vi "FTW-Scripter-LoadScript.vi"(0 "FTW Actor Connector In":refnum<class "FTW-ActorConnector.lvclass">, 7 "Script":string, 11 "error in (no error)":errorcluster) -> (4 "FTW Actor Connector":refnum<class "FTW-ActorConnector.lvclass">, 8 "My Message Response":bool, 14 "Roundtrip Time":dbl format="%.6f sec", 15 "error out":errorcluster)   [LabVIEW 2015]
uses:
  source/actor/Connector/FTW-ActorConnector.lvclass
  source/JSON/core/FTW-JSON-Core-EncodingFlags.vi
  source/JSON/FTW-JSON-Parse.vi
  source/Reflection/FTW-Reflection-Type.vi
  source/CodeGen/JSON Deserialize/FTW-JSON-Core-GetFlattenedValue.vi
  source/CodeGen/JSON Deserialize/FTW-JSON-Deserialize.xnode
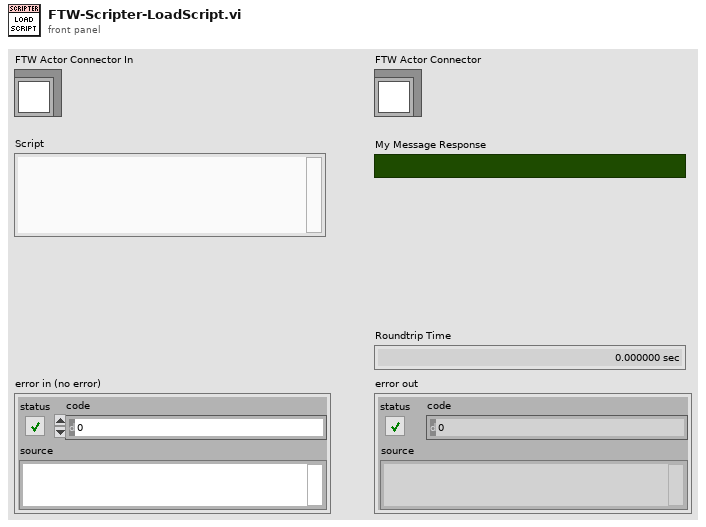
[diagram p1: front panel]
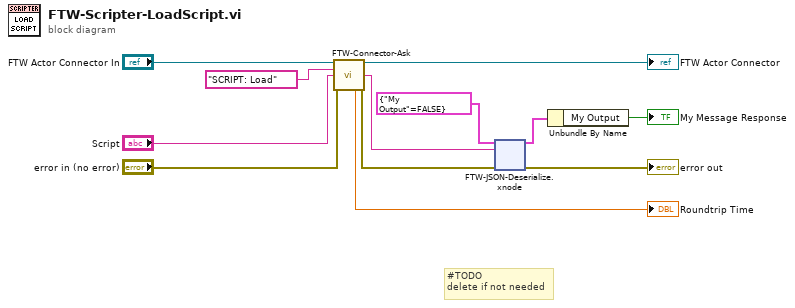
[diagram p0: block diagram]
diagram:
  # "#TODO\ndelete if not needed"
  n1 = call "FTW-Connector-Ask.vi"("FTW Actor Connector"="FTW Actor Connector In", "Request Header"="SCRIPT: Load", "Request Body"="Script", "error in"="error in (no error)") -> ("FTW Actor Connector out"=→"FTW Actor Connector":refnum<class "FTW-ActorConnector.lvclass">, "Response Body"=w5:string, "Roundtrip Time"=→"Roundtrip Time":dbl, "error out"=w8:errorcluster)  [unwired: 6 in, 2 out]
  n2 = xnode "FTW-JSON-Deserialize.xnode"("Type and Defaults"=cluster{"My Output":bool} {"My Output"=FALSE}, "JSON String"=w5, "error in"=w8) -> ("Values"=w3:cluster{"My Output":bool}, "error out"=→"error out":errorcluster)
  n3 = Unbundle By Name(w3) -> ("My Output"=→"My Message Response":bool)
